vi "t.vi"(11 "待处理字符串":string) -> (3 "finally":string[][](array[string]))   [LabVIEW 2017]
uses:
  <vilib>/regexp/Match Regular Expression.xnode
panel:
  out "结果字符串":string
  out "ADC":string
  out "ADC":string[](array[string])
  out "V":string[](array[string])
  out "CH":string[](array[string])
  out "V":string
  out "CH":string
  out "匹配之后":string
  out "匹配之前":string
  out "所有匹配":string
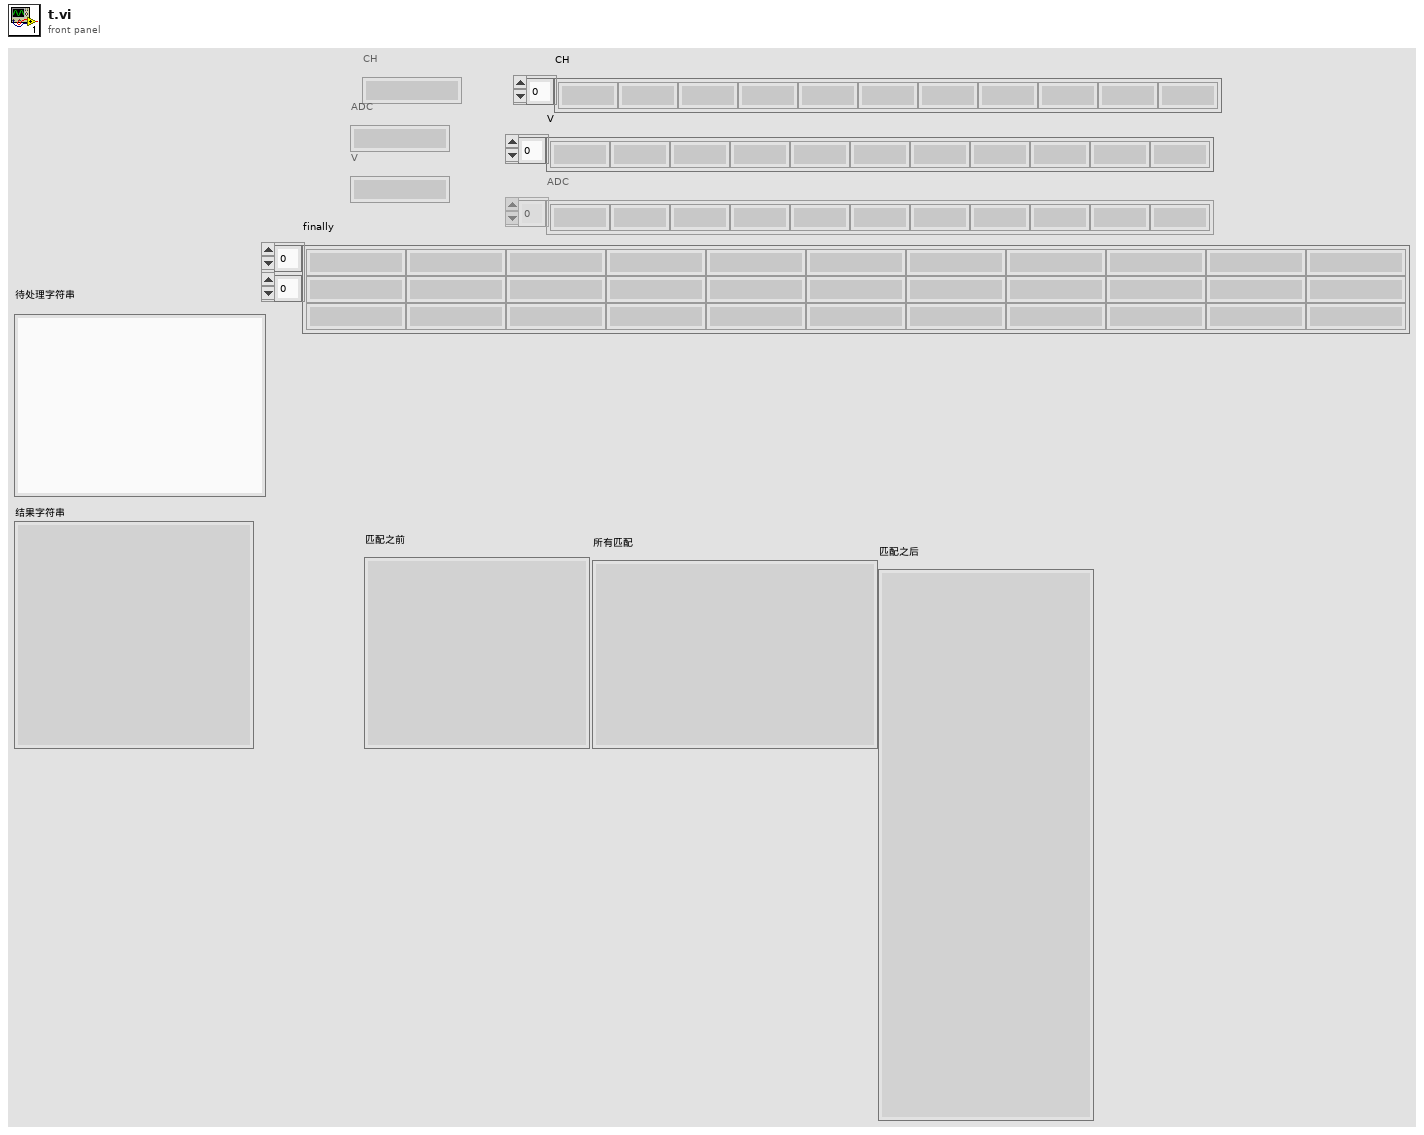
[diagram p1: front panel]
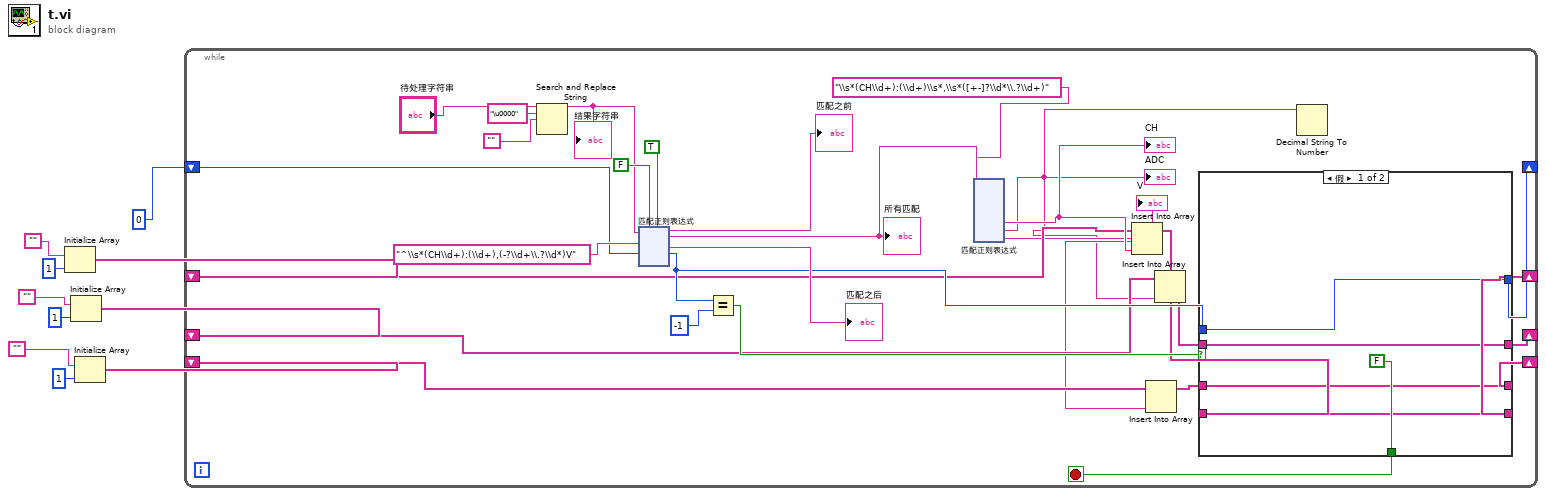
[diagram p0: block diagram]
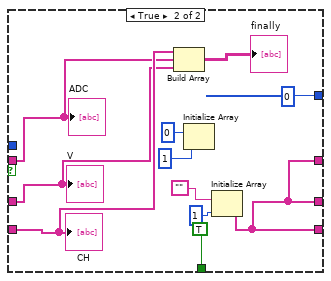
[diagram p2: hidden frame]
diagram:
  n1 = Initialize Array("", 1 ("维数大小")) -> (w9:string[])
  n2 = Initialize Array("", 1 ("维数大小")) -> (w5:string[])
  n3 = Initialize Array("", 1 ("维数大小")) -> (w3:string[])
  n4 = while {
    shift-right: [w30] -> _
    shift-left: 0 -> [w29]
    shift-right: [w17] -> _
    shift-left: w9 -> [w25]
    shift-right: [w19] -> _
    shift-left: w5 -> [w24]
    shift-right: [w21] -> _
    shift-left: w3 -> [w23]
    stop <- w32 stop-if-true
    n5 = Search and Replace String(input string="待处理字符串", search string="\u0000" ("搜索字符串"), replace string="") -> (result string=w13:string)  [unwired: 5 in, 3 out]
    "结果字符串" <- w13
    n6 = xnode "匹配正则表达式"("输入字符串"=w13, "正则表达式"="^\\s*(CH\\d+):(\\d+),(-?\\d+\\.?\\d*)V", "偏移量(0)"=w29, "忽略大小写？(F)"=FALSE, "多行？<B><B>(F)</B></B>"=TRUE) -> ("匹配之前"=→"匹配之前":string, "所有匹配"=w28:string, "匹配之后"=→"匹配之后":string, "匹配后偏移量"=w31:i32)  [unwired: 1 in, 1 out]
    "所有匹配" <- w28
    n7 = Equal?(x=w31, y=-1) -> (x = y?=w33:bool)
    n8 = xnode "匹配正则表达式"("输入字符串"=w28, "正则表达式"="\\s*(CH\\d+):(\\d+)\\s*,\\s*([+-]?\\d*\\.?\\d+)") -> ("子匹配 1"=w26:string, "子匹配 2"=w15:string, "子匹配 3"=w16:string)  [unwired: 4 in, 5 out]
    "CH" <- w26
    "V" <- w16
    "ADC" <- w15
    n9 = Insert Into Array(array=w25, new element=w26) -> (w18:string[])  [unwired: 1 in]
    n10 = Insert Into Array(array=w23, new element=w16) -> (w22:string[])  [unwired: 1 in]
    n11 = Insert Into Array(array=w24, new element=w15) -> (w20:string[])  [unwired: 1 in]
    n12 = case shown="假" w33 {
      tunnel: [FALSE TRUE] -> w32
      tunnel: w31 -> [w162 _]
      tunnel: [w162 0] -> w30
      tunnel: w22 -> [w160 w164]
      tunnel: [w160 w166] -> w21
      tunnel: w20 -> [w159 w165]
      tunnel: [w159 w166] -> w19
      tunnel: w18 -> [w158 w167]
      tunnel: [w158 w166] -> w17
      frame False {
      }
      frame True {
        n13 = Build Array(w167, w165, w164) -> (→"finally":string[][])
        n14 = Initialize Array(0 ("元素"), 1 ("维数大小")) -> ()  [unwired: 1 out]
        n15 = Initialize Array("", 1 ("维数大小")) -> (w166:string[])
        "CH" <- w167
        "V" <- w164
        "ADC" <- w165
      }
    }
    n16 = Decimal String To Number(string=w15) -> ()  [unwired: 2 in, 2 out]
  }
